vi "Encode packed uint64.vi"(7 "Field Number":i32, 10 "uint64":u64[](array[numeric]), 11 "Buffer in":u8[](array[numeric]) format="%.0x") -> (3 "Buffer":u8[](array[numeric]) format="%.0x")   [LabVIEW 2020, in "LV-Proto.lvlib"]
uses:
  LV-Proto.lvlib
  Wire Type.ctl
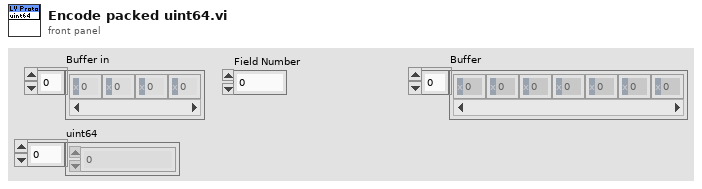
[diagram p1: front panel]
types:
  T1 = typedef "LV-Proto.lvlib/Wire Type.ctl" = enum8{"VARINT", "I64", "LEN", "SGROUP (Deprecated)", "EGROUP (Deprecated)", "I32"}
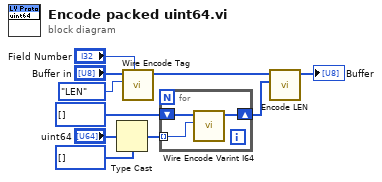
[diagram p0: block diagram]
diagram:
  n1 = Type Cast(type=i64[] [], x="uint64") -> (*(type *) &x=w2:i64[])
  n2 = call "Wire Encode Tag.vi"("Field Number"="Field Number", "Wire Type"=Wire_Type."LEN", "Buffer in"="Buffer in") -> ("Buffer"=w7:u8[])  [unwired: 8 in]
  n3 = for {
    shift-right: [w11] -> w3
    shift-left: u8[] [] ("Buffer") -> [w13]
    tunnel: w2 -> [w12] mode=indexing
    n4 = call "Wire Encode Varint I64.vi"("I64"=w12, "Buffer in"=w13) -> ("Buffer"=w11:u8[])  [unwired: 9 in]
  }
  n5 = call "Encode LEN.vi"("Data"=w3, "Buffer in"=w7) -> ("Buffer"=→"Buffer":u8[])  [unwired: 9 in]
